vi "TCS_Tx.vi"() -> ()   [LabVIEW 2018]
uses:
  Stream/Stream.lvclass
  RxTx/RxTx.lvclass
panel:
  in  "RxTx.lvclass":refnum<class "RxTx.lvclass">
  in  "Stream.lvclass":refnum<class "Stream.lvclass">
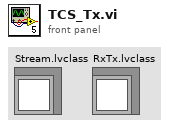
[diagram p1: front panel]
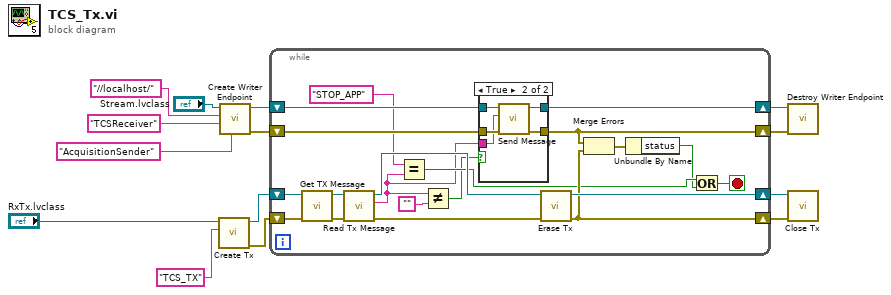
[diagram p0: block diagram]
diagram:
  n1 = call "Create Tx.vi"("Writer Name"="TCS_TX" ("Reader Name"), "RxTx in"="RxTx.lvclass") -> ("error out"=w12:errorcluster, "RxTx out"=w13:refnum<class "RxTx.lvclass">)  [unwired: 8 in]
  n2 = call "Create Writer Endpoint.vi"("writer name"="AcquisitionSender" ("reader name"), "reader name"="TCSReceiver", "IP"="//localhost/" ("Reader Name"), "Stream in"="Stream.lvclass") -> ("error out"=w6:errorcluster, "Stream out"=w8:refnum<class "Stream.lvclass">)  [unwired: 6 in]
  n3 = while {
    shift-right: [w26] -> w5
    shift-left: w6 -> [w28]
    shift-right: [w27] -> w14
    shift-left: w8 -> [w29]
    shift-right: [w21] -> w9
    shift-left: w12 -> [w30]
    shift-right: [w23] -> w10
    shift-left: w13 -> [w31]
    stop <- w18 stop-if-true
    n4 = call "Get TX Message.vi"("error in (no error)"=w30, "RxTx in"=w31) -> ("error out"=w33:errorcluster, "RxTx out"=w32:refnum<class "RxTx.lvclass">)  [unwired: 8 in]
    n5 = call "Read Tx Message.vi"("error in (no error)"=w33, "RxTx in"=w32) -> ("error out"=w22:errorcluster, "Tx Message"=w16:string, "RxTx out"=w24:refnum<class "RxTx.lvclass">)  [unwired: 7 in]
    n6 = Equal?(x="STOP_APP", y=w16) -> (x = y?=w20:bool)
    n7 = Not Equal?(x=w16, y="") -> (x != y?=w15:bool)
    n8 = case shown="True" w15 {
      tunnel: w29 -> [w36 w41]
      tunnel: w28 -> [w35 w40]
      tunnel: [w36 w39] -> w27
      tunnel: w16 -> [_ w38]
      tunnel: [w35 w37] -> w26
      frame False {
      }
      frame True {
        n9 = call "Send Message.vi"("error in (no error)"=w40, "Message"=w38, "Stream in"=w41) -> ("error out"=w37:errorcluster, "Stream out"=w39:refnum<class "Stream.lvclass">)  [unwired: 7 in]
      }
    }
    n10 = call "Erase Tx.vi"("error in (no error)"=w22, "RxTx in"=w24) -> ("error out"=w21:errorcluster, "RxTx out"=w23:refnum<class "RxTx.lvclass">)  [unwired: 8 in]
    n11 = Merge Errors(w26, w21) -> (w34:errorcluster)
    n12 = Unbundle By Name(w34) -> ("status"=w19:bool)
    n13 = Or(x=w20, y=w19) -> (x .or. y?=w18:bool)
  }
  n14 = call "Destroy Writer Endpoint.vi"("error in (no error)"=w5, "Stream in"=w14) -> ()  [unwired: 8 in, 2 out]
  n15 = call "Close Tx.vi"("error in (no error)"=w9, "RxTx in"=w10) -> ()  [unwired: 8 in, 2 out]
